vi "RSZVB Get Port Waveguide Attenuator.vi"(7 "Waveguide Attenuator (Mechanical)":i32(ring) items=["Mechanical", "Electronic"], 8 "error in (no error)":errorcluster {"code" format="%.0x"}, 9 "Port (1)":i32=1, 10 "Channel (1)":i32=1, 11 "VISA session":refnum<visa-resource-name>) -> (0 "error out":errorcluster {"code" format="%.0x"}, 2 "Attenuation":dbl format="%^.3e", 3 "dup VISA session":refnum<visa-resource-name>)   [LabVIEW 2011]
doc: "This VI returns the waveguide attenuator type of the converter port <Pt> and attenuation for a converter with electronic or mechanical attenuators at port <Pt>.\n\nRemote-control command(s):\nSOURce<Ch>:POWer<Pt>:CONVerter:TRANsfer:ELECtronic:MATTenuation?\nSOURce<Ch>:POWer<Pt>:CONVerter:TRANsfer:MECHanical:ATTenuation?"
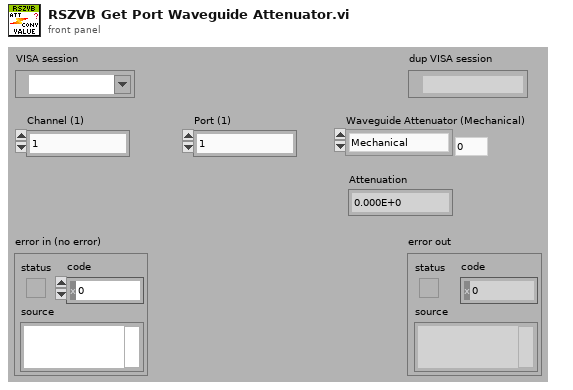
[diagram p1: front panel]
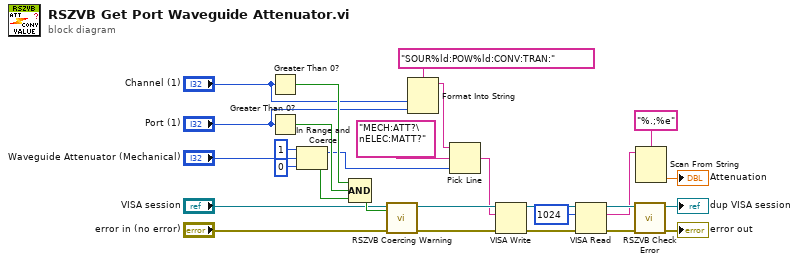
[diagram p0: block diagram]
diagram:
  n1 = Greater Than 0?(x="Channel (1)") -> (x > 0?=w24:bool)
  n2 = Greater Than 0?(x="Port (1)") -> (x > 0?=w22:bool)
  n3 = In Range and Coerce(upper limit=1, x="Waveguide Attenuator (Mechanical)", lower limit=0) -> (coerced(x)=w20:i32, In Range?=w27:bool)
  n4 = Compound Arithmetic op=AND(w24, w22, w27) -> (w26:bool)
  n5 = call "RSZVB Coercing Warning.vi"("In Range?"=w26, "error in (no error)"="error in (no error)", "VISA session"="VISA session") -> ("error out"=w12:errorcluster, "dup VISA session"=w13:refnum<visa-resource-name>)  [unwired: 7 in]
  n6 = Format Into String(format string="SOUR%ld:POW%ld:CONV:TRAN:", "Channel (1)", "Port (1)") -> (resulting string=w14:string)  [unwired: 2 in, 1 out]
  n7 = Pick Line(string ("")=w14, multi-line string="MECH:ATT?\nELEC:MATT?", line index=w20) -> (output string=w11:string)
  n8 = VISA Write(VISA resource name=w13, write buffer=w11, error in (no error)=w12) -> (VISA resource name out=w8:refnum<visa-resource-name>, error out=w7:errorcluster)  [unwired: 1 out]
  n9 = VISA Read(VISA resource name=w8, byte count=u32 1024, error in (no error)=w7) -> (VISA resource name out=w9:refnum<visa-resource-name>, read buffer=w3:string, error out=w6:errorcluster)  [unwired: 1 out]
  n10 = call "RSZVB Check Error.vi"("error in (no error)"=w6, "VISA session"=w9) -> ("error out"=→"error out":errorcluster, "dup VISA session"=→"dup VISA session":refnum<visa-resource-name>)  [unwired: 8 in]
  n11 = Scan From String(format string="%.;%e", input string=w3) -> (output 1=→"Attenuation":dbl)  [unwired: 3 in, 3 out]
